vi "Parse Message.vi"(11 "Body":string) -> (1 "found?":bool, 2 "Remaining string":string, 3 "Message":T1)   [LabVIEW 2015, in "NI_Azure_Queue.lvlib"]
uses:
  NI_Azure_Queue.lvlib
  Message.ctl
  XML Parsing/NI_Azure_XML Parsing.lvlib
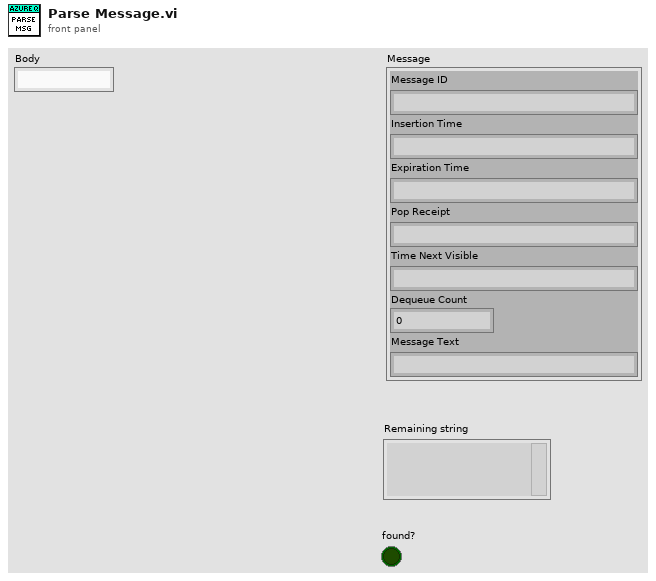
[diagram p1: front panel]
types:
  T1 = typedef "NI_Azure_Queue.lvlib/Message.ctl" = cluster{"Message ID":string, "Insertion Time":string, "Expiration Time":string, "Pop Receipt":string, "Time Next Visible":string, "Dequeue Count":i32, "Message Text":string}
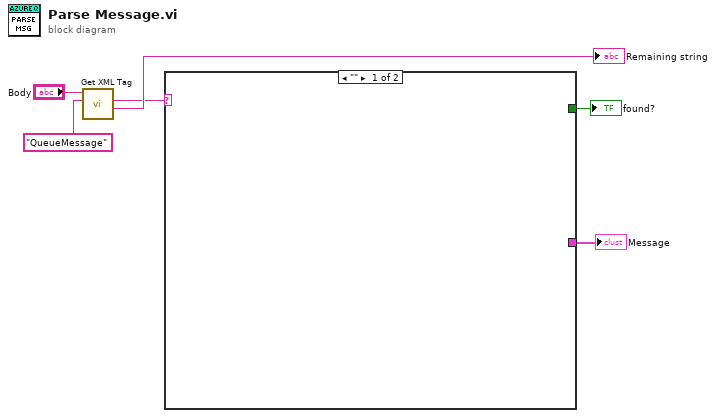
[diagram p0: block diagram]
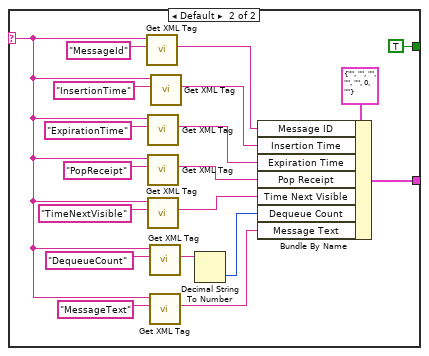
[diagram p2: hidden frame]
diagram:
  n1 = call "Get XML Tag.vi"("Tag name"="QueueMessage", "XML String in"="Body") -> ("Remaining string"=→"Remaining string":string, "Tag value"=w2:string)  [unwired: 5 in, 3 out]
  n2 = case shown="\"\"" w2 {
    selector: w2 -> [_ w8]
    tunnel: [_ w17] -> w6
    tunnel: [_ TRUE] -> w1
    frame "" {
    }
    frame Default {
      n3 = call "Get XML Tag.vi"("Tag name"="MessageId", "XML String in"=w8) -> ("Tag value"=w18:string)  [unwired: 5 in, 4 out]
      n4 = call "Get XML Tag.vi"("Tag name"="ExpirationTime", "XML String in"=w8) -> ("Tag value"=w20:string)  [unwired: 5 in, 4 out]
      n5 = call "Get XML Tag.vi"("Tag name"="PopReceipt", "XML String in"=w8) -> ("Tag value"=w21:string)  [unwired: 5 in, 4 out]
      n6 = call "Get XML Tag.vi"("Tag name"="TimeNextVisible", "XML String in"=w8) -> ("Tag value"=w22:string)  [unwired: 5 in, 4 out]
      n7 = call "Get XML Tag.vi"("Tag name"="DequeueCount", "XML String in"=w8) -> ("Tag value"=w24:string)  [unwired: 5 in, 4 out]
      n8 = call "Get XML Tag.vi"("Tag name"="MessageText", "XML String in"=w8) -> ("Tag value"=w23:string)  [unwired: 5 in, 4 out]
      n9 = call "Get XML Tag.vi"("Tag name"="InsertionTime", "XML String in"=w8) -> ("Tag value"=w19:string)  [unwired: 5 in, 4 out]
      n10 = Decimal String To Number(string=w24) -> (number=w25:i32)  [unwired: 2 in, 1 out]
      n11 = Bundle By Name(cluster=T1 {"Message ID"="", "Insertion Time"="", "Expiration Time"="", "Pop Receipt"="", "Time Next Visible"="", "Dequeue Count"=0, "Message Text"=""} ("Message"), "Message ID"=w18, "Insertion Time"=w19, "Expiration Time"=w20, "Pop Receipt"=w21, "Time Next Visible"=w22, "Dequeue Count"=w25, "Message Text"=w23) -> (w17:T1)
    }
  }
  "Message" <- w6
  "found?" <- w1
